vi "errorException.vi"(8 "error in (no error)":errorcluster) -> (0 "error IO":errorcluster)   [LabVIEW 2015, in "pdbm_task_route.lvlib"]
uses:
  pdbm_task_route.lvlib
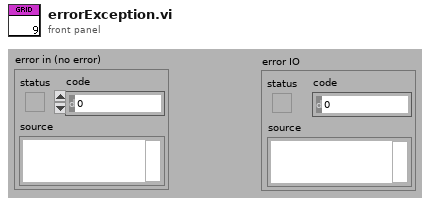
[diagram p1: front panel]
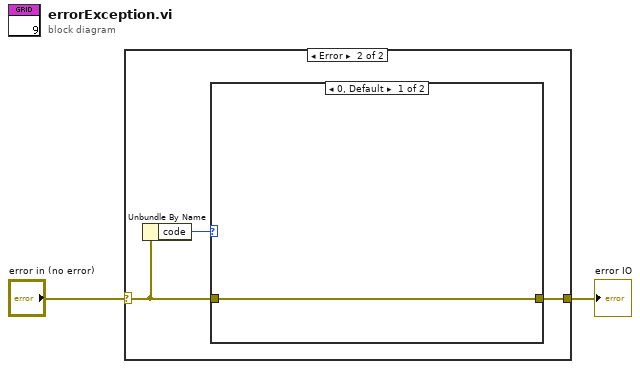
[diagram p0: block diagram]
diagram:
  n1 = case shown="Error" "error in (no error)" {
    selector: "error in (no error)" -> [w3 w5]
    tunnel: [w3 w4] -> w1
    frame No Error {
    }
    frame Error {
      n2 = Unbundle By Name(w5) -> ("code"=w6:i32)
      n3 = case shown="0, Default" w6 {
        tunnel: w5 -> [w7 _]
        tunnel: [w7 _] -> w4
        frame 0, Default {
        }
        frame 1 {
        }
      }
    }
  }
  "error IO" <- w1
